vi "Driver Variables_MFP3D_Lucy.vi"() -> ()   [LabVIEW 2019]
panel:
  in  "channel 2":tag
  in  "channel 1":tag
  in  "abort lithography?":bool
  out "lithography running?":bool
  out "tip engaged?":bool
  out "litho comm":T1
  in  "Inkscape ratio":dbl
  in  "Amplifier Setting":dbl=-10.0
  in  "Read Tip Voltage":dbl
  in  "Old Y Offset":dbl
  in  "Old X Offset":dbl
  in  "Y Offset":dbl
  in  "X Offset":dbl
  in  "Old Image Width":dbl=40.0
  in  "Old Image Height":dbl=40.0
  in  "Image Width":dbl=40.0
  in  "Image Height":dbl=40.0
  in  "Old RGB Value":u32
  in  "RGB Value":u32
  in  "Old Visible":bool=TRUE
  in  "Visible":bool=TRUE
  in  "Old Center of Vision":string="(0,0,0)"
  in  "Center of Vision":string="(0,0,0)"
  in  "Old Wire Width":dbl=0.01
  in  "Old Voltage":dbl
  in  "Old Y":dbl=15.0
  in  "Old X":dbl=15.0
  in  "Wire Width":dbl=0.1
  in  "Voltage":dbl
  in  "Y":dbl=7.418777765268947
  in  "X":dbl=26.509542
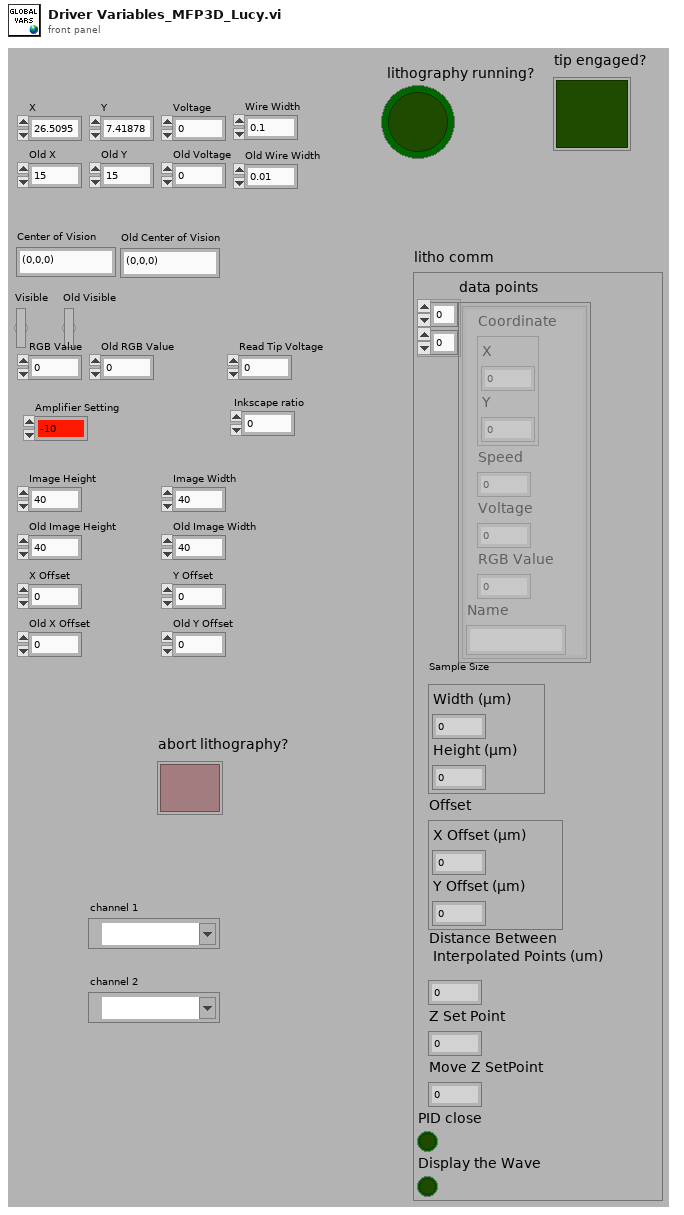
[diagram p1: front panel]
types:
  T1 = cluster{"data points":cluster{"Coordinate":cluster{"X":dbl, "Y":dbl}, "Speed":dbl, "Voltage":dbl, "RGB Value":i32, "Name":string}[][], "Sample Size":cluster{"Width (µm)":dbl, "Height (µm)":dbl}, "Offset":cluster{"X Offset (µm)":dbl, "Y Offset (µm)":dbl}, "Distance Between\n Interpolated Points (um)":dbl, "Z Set Point":dbl, "Move Z SetPoint":dbl, "PID close":bool, "Display the Wave":bool}
diagram:
